vi "FLUSHALL.vi"(0 "refnum in":refnum<vi>, 11 "error in":errorcluster) -> (4 "refnum out":refnum<vi>, 6 "Data":T1, 15 "error out":errorcluster)   [LabVIEW 2023]
uses:
  SubVIs/Controls/redis-data.ctl
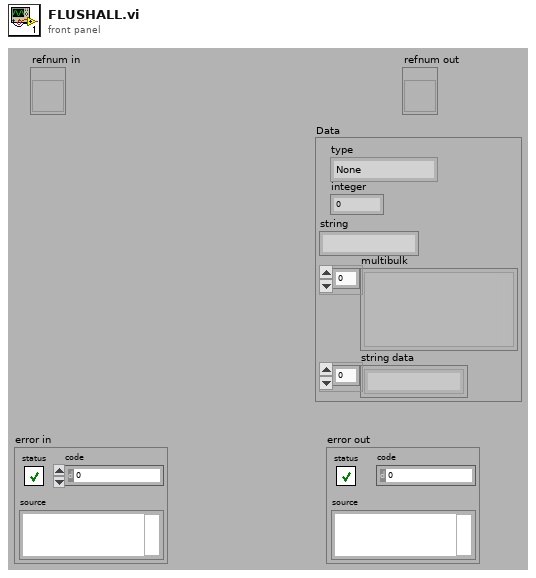
[diagram p1: front panel]
types:
  T1 = typedef "redis-data.ctl" = cluster{"type":enum16{"None", "Error", "Status", "Nil", "Integer", "String", "Multibulk"}, "integer":i64, "string":string, "multibulk":variant[], "string data":string[]}
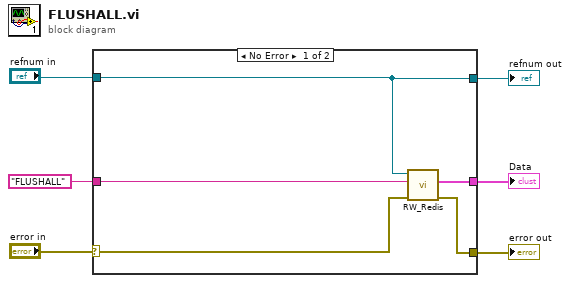
[diagram p0: block diagram]
diagram:
  n1 = case shown="No Error" "error in" {
    selector: "error in" -> [w11 w13]
    tunnel: "FLUSHALL" -> [w7 _]
    tunnel: "refnum in" -> [w8 w12]
    tunnel: [w10 w13] -> w4
    tunnel: [w9 _] -> w1
    tunnel: [w8 w12] -> w2
    frame No Error {
      n2 = call "RW_Redis.vi"("error in"=w11, "command"=w7, "TCP session in"=w8) -> ("error out"=w10:errorcluster, "Data"=w9:T1)  [unwired: 6 in, 1 out]
    }
    frame Error {
    }
  }
  "error out" <- w4
  "refnum out" <- w2
  "Data" <- w1
